vi "Angulo de encoder.vi"(8 "error in (no error)":errorcluster, 11 "Input angle":dbl) -> (0 "error out":errorcluster, 3 "Output angle":dbl)   [LabVIEW 2018]
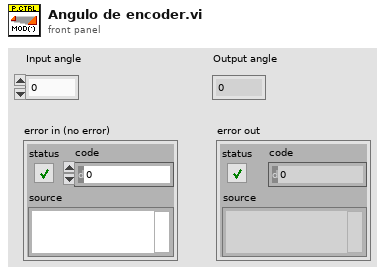
[diagram p1: front panel]
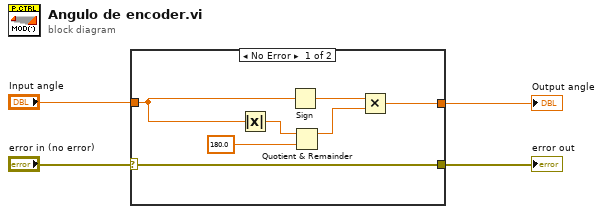
[diagram p0: block diagram]
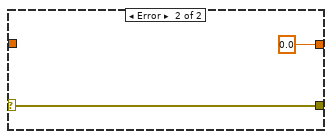
[diagram p2: hidden frame]
diagram:
  n1 = case shown="No Error" "error in (no error)" {
    selector: "error in (no error)" -> [w5 w12]
    tunnel: [w11 0.0] -> w4
    tunnel: "Input angle" -> [w8 _]
    tunnel: [w5 w12] -> w1
    frame No Error {
      n2 = Absolute Value(x=w8) -> (abs(x)=w7:dbl)
      n3 = Sign(1:w8) -> (0:w9:dbl)
      n4 = Quotient & Remainder(x=w7, y=180.0) -> (x-y*floor(x/y)=w10:dbl)  [unwired: 1 out]
      n5 = Multiply(x=w9, y=w10) -> (x*y=w11:dbl)
    }
    frame Error {
    }
  }
  "Output angle" <- w4
  "error out" <- w1
